vi "asset.data_source_type_at.vi"(8 "error in":errorcluster, 11 "object_in":refnum<class "Asset.lvclass">) -> (0 "error out":errorcluster, 3 "object_out":refnum<class "Asset.lvclass">)   [LabVIEW 2020, in "Asset.lvclass"]
doc: "Returns the kind (dataset, video, or connection) of the data source at the given index."
uses:
  Asset.lvclass
  Asset.lvclass/Asset.ctl
  client.lvlib
panel:
  out "function return":i32
  out "out_type out":i32
  in  "index":i32
  in  "out_type":i32
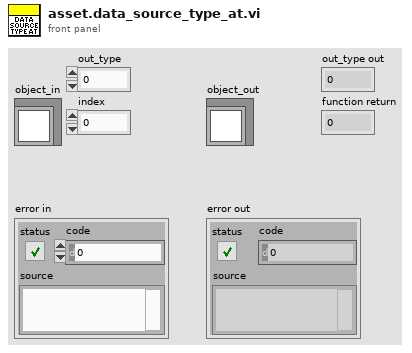
[diagram p1: front panel]
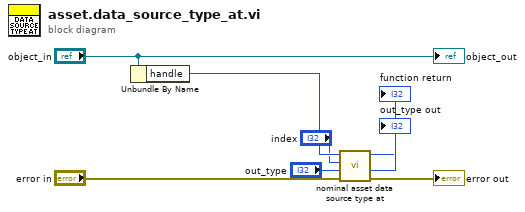
[diagram p0: block diagram]
diagram:
  n1 = Unbundle By Name("object_in") -> ("handle"=w6:i32)
  n2 = call "nominal asset data source type at.vi"("error in (no error)"="error in", "out_type"="out_type", "index"="index", "asset"=w6) -> ("error out"=→"error out":errorcluster, "out_type out"=→"out_type out":i32, "function return"=→"function return":i32)  [unwired: 5 in]
  "object_out" <- "object_in"
